vi "Multiple Waveforms.vi"(8 "error in (no error)":errorcluster, 11 "Multiple Waveforms":waveform(dbl)[](array[waveform])) -> (0 "error out":errorcluster, 2 "2D Array":dbl[][](array[numeric]))   [LabVIEW 2016]
doc: "This instance will convert a 1D array of waveforms to a 2D array of doubles. The first column of the resulting 2D array will be the time data of the first waveform, indexed at 0."
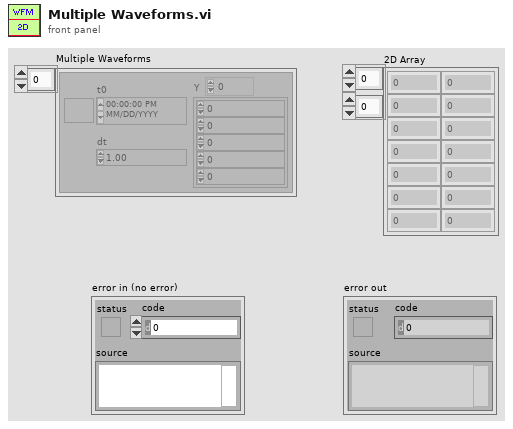
[diagram p1: front panel]
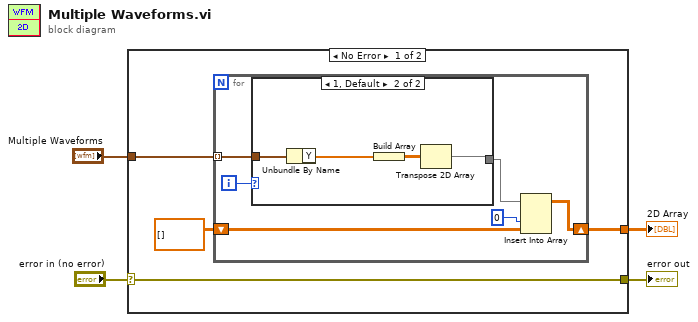
[diagram p0: block diagram]
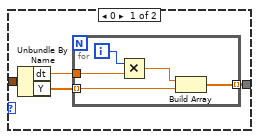
[diagram p2: hidden frame]
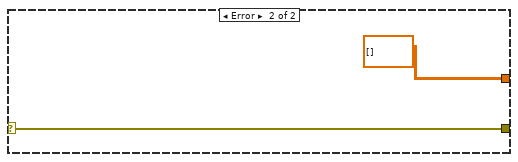
[diagram p3: hidden frame]
diagram:
  n1 = case shown="No Error" "error in (no error)" {
    selector: "error in (no error)" -> [w6 w29]
    tunnel: [w8 dbl[][] []] -> w4
    tunnel: "Multiple Waveforms" -> [w7 _]
    tunnel: [w6 w29] -> w2
    frame No Error {
      n2 = for {
        tunnel: w7 -> [w14] mode=indexing
        shift-right: [w10] -> w8
        shift-left: dbl[][] [] -> [w11]
        i -> [w13]
        n3 = case shown="1, Default" w13 {
          tunnel: [w16 w24] -> w12
          tunnel: w14 -> [w15 w27]
          frame 0 {
            n4 = Unbundle By Name(w15) -> ("dt"=w18:dbl, "Y"=w17:dbl[])
            n5 = for {
              tunnel: w18 -> [w23]
              tunnel: w17 -> [w21] mode=indexing
              tunnel: [w19] -> w16 mode=indexing
              i -> [w22]
              n6 = Multiply(x=w22, y=w23) -> (x*y=w20:dbl)
              n7 = Build Array(w20, w21) -> (w19:dbl[])
            }
          }
          frame 1, Default {
            n8 = Unbundle By Name(w27) -> ("Y"=w26:dbl[])
            n9 = Build Array(w26) -> (w25:dbl[][])
            n10 = Transpose 2D Array(2D array=w25) -> (transposed array=w24:dbl[][])
          }
        }
        n11 = Insert Into Array(array=w12, index (col)=0 ("disabled index (col)"), new element=w11) -> (w10:dbl[][])  [unwired: 1 in]
      }
    }
    frame Error {
    }
  }
  "2D Array" <- w4
  "error out" <- w2
